vi "Vision Processing.vi"(4 "error in (no error)":errorcluster, 7 "Image Size":T1=enum."320x240") -> ()   [LabVIEW 2015]
doc: "This VI runs in parallel to other tasks. It gets images from the camera, processes them for color or shape and use that information to affect robot behavior."
uses:
  Support Vision Code/Camera Types.ctl
  <vilib>/Rock Robotics/WPI/Camera/WPI_CameraImageSize.ctl
  <userlib>/836-Library/System/QCP Support Code/QCP_Get_DBL.vi
  <userlib>/836-Library/System/QCP Support Code/QCP_Get_STR.vi
  <vilib>/Rock Robotics/Network Tables/NT Read Boolean.vi
  <userlib>/836-Library/System/QCP Support Code/QCP_Set_DBL.vi
  <vilib>/Rock Robotics/Network Tables/NT Write String.vi
  <vilib>/Rock Robotics/Network Tables/NT Write Number.vi
  <vilib>/Rock Robotics/Network Tables/NT Write Boolean.vi
  <vilib>/Rock Robotics/Network Tables/NT Read Number.vi
  <vilib>/Rock Robotics/Network Tables/NT Read String.vi
  Robot Global Data.vi
  <vilib>/vision/NI_Vision_Development_Module.lvlib
panel:
  out "Right Target":dbl
  out "Left Target":dbl
  out "Target Angle":dbl
  in  "Sideways Camera":bool
  in  "Boresight":dbl format="%#_13g"
  out "Found Targets":T2(array[cluster])=[{"Bounding box"={"left"=112.0, "top"=150.0, "right"=139.0, "bottom"=174.0}, "Aspect Ratio"=70.3125, "Area to CH"=96.83972911963883, "X Mask"=77.77777777777779, "Y Mask"=70.83333333333334, "Moment"=69.2156660279794}]
  out "FPS":dbl=5.212996497577636
  out "Qualified Particles":i32=2
  in  "Score Threshold":dbl=70.0
  in  "Aspect Fudge Factor":dbl=1.0
  in  "Min Score Threshold":dbl=75.0
  in  "Camera Type":T3=enum."MS HD3000 square"
  in  "Emphasize Limit Tests":bool
  out "Masked":T4(plugin-control)
  out "Original Image":T4(plugin-control)
  in  "Display Original":bool=TRUE
  out "Sorted Particle Scores":T5(array[cluster])=[{"Rectangle px"={"Numeric"=112.0, "Numeric 2"=150.0, "Numeric 3"=139.0, "Numeric 5"=174.0}, "Aspect Ratio"=70.3125, "Area to CH"=96.83972911963883, "X"=77.77777777777779, "Y"=70.83333333333334, "Moment Factor"=69.2156660279794}] {"Moment Factor" format="%#_3g"; "Aspect Ratio" format="%#_3g"; "Area to CH" format="%#_3g"; "X" format="%#_3g"; "Y" format="%#_3g"}
  out "Detected Targets":T6(array[cluster])=[{"Distance (ft)"=26.324888830153935, "Center"={-0.3966346153846153, -0.35}, "Normalized Rect"={"Numeric"=-0.46153846153846145, "Numeric 2"=-0.25, "Numeric 3"=-0.33173076923076916, "Numeric 5"=-0.44999999999999996}}] {"Normalized Rect"."Numeric 5" format="%#_2g"; "Normalized Rect"."Numeric 3" format="%#_2g"; "Normalized Rect"."Numeric 2" format="%#_2g"; "Normalized Rect"."Numeric" format="%#_2g"}
  in  "LED Color":T7={"Hue"={152.2312396148097, 250.0}, "Sat"={154.82142857142858, 255.0}, "Val"={100.17857142857143, 255.0}} {"Hue" scale=0.0..255.0 scale format="%#_3g"}
  # "Density Profile"
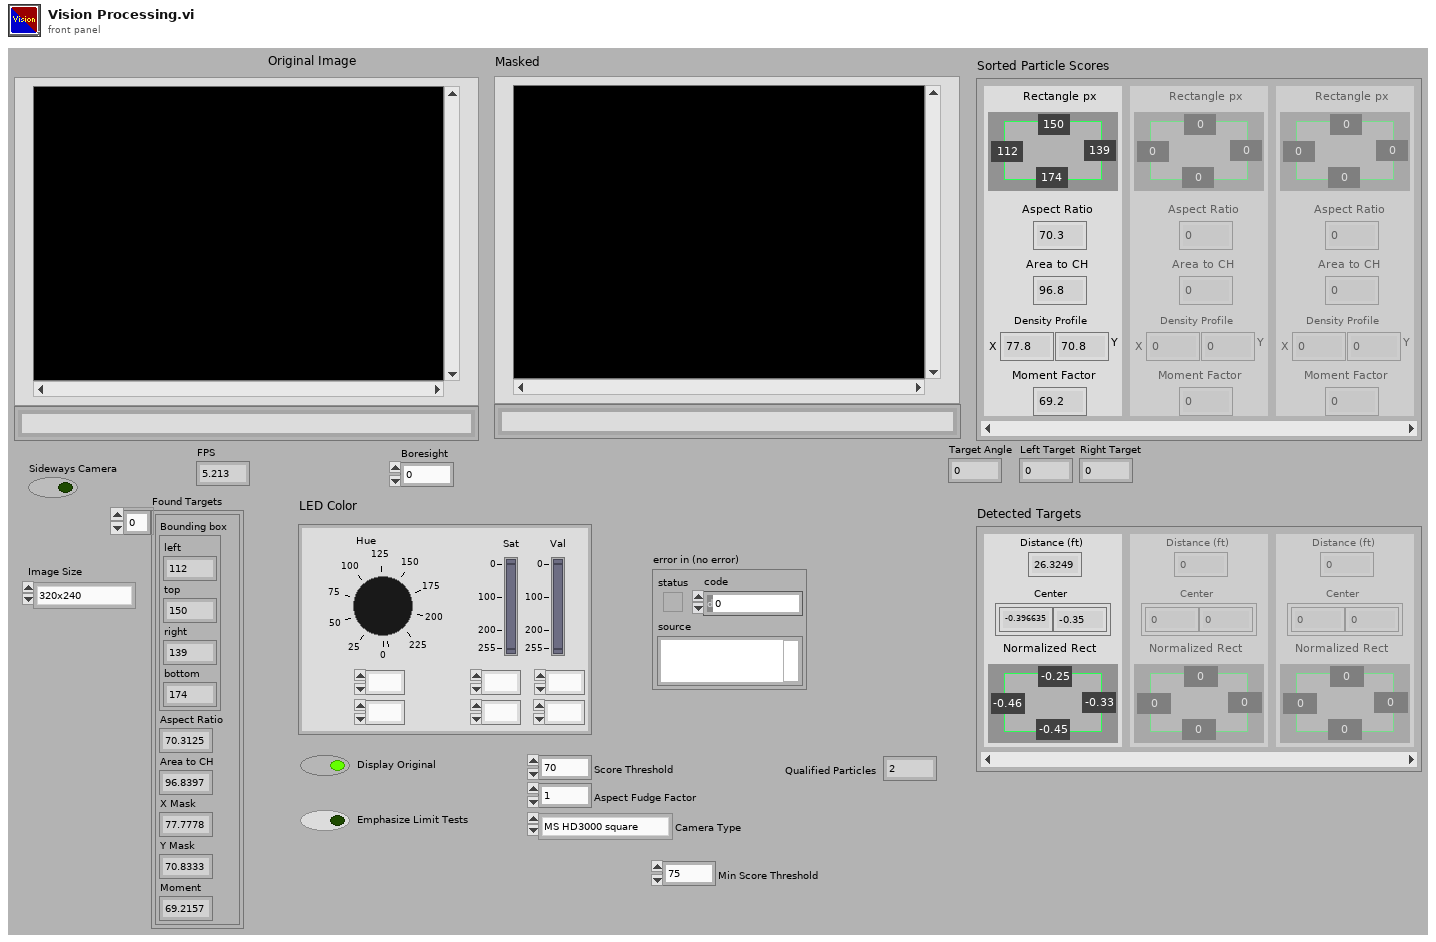
[diagram p1: front panel]
types:
  T1 = typedef "WPI_CameraImageSize.ctl" = enum16{"640x480", "320x240", "160x120", "Custom"}
  T2 = cluster{"Bounding box":cluster{"left":dbl, "top":dbl, "right":dbl, "bottom":dbl}, "Aspect Ratio":dbl, "Area to CH":dbl, "X Mask":dbl, "Y Mask":dbl, "Moment":dbl}[]
  T3 = typedef "Camera Types.ctl" = enum16{"206", "1011", "1013", "MS HD3000 square", "MS HD3000 640x480"}
  T4 = typedef "IMAQ Image.ctl" = refnum<image>
  T5 = cluster{"Rectangle px":cluster{"Numeric":dbl, "Numeric 2":dbl, "Numeric 3":dbl, "Numeric 5":dbl}, "Aspect Ratio":dbl, "Area to CH":dbl, "X":dbl, "Y":dbl, "Moment Factor":dbl}[]
  T6 = cluster{"Distance (ft)":dbl, "Center":cluster{dbl, dbl}, "Normalized Rect":cluster{"Numeric":dbl, "Numeric 2":dbl, "Numeric 3":dbl, "Numeric 5":dbl}}[]
  T7 = cluster{"Hue":cluster{dbl, dbl}, "Sat":cluster{dbl, dbl}, "Val":cluster{dbl, dbl}}
  T8 = typedef "Particle Parameters" = i32
  T9 = typedef "Image Type" = u32
  T10 = typedef "QCP Data Block.ctl" = refnum<data-value>
  T11 = typedef "WPI_CameraDevRef.ctl" = cluster{"Camera Address":string, "CameraStatus":errorcluster}
  T12 = cluster{cluster{"Value Out":dbl, "Value Out":dbl}, cluster{"Value Out":dbl, "Value Out":dbl}, cluster{"Value Out":dbl, "Value Out":dbl}}
  T13 = cluster{"Rectangle":cluster{"Numeric":dbl, "Numeric 2":dbl, "Numeric 3":dbl, "Numeric 5":dbl}, "L":dbl, "Area to CH":dbl, "X":dbl, "Y":dbl, "Moment Factor":dbl}[]
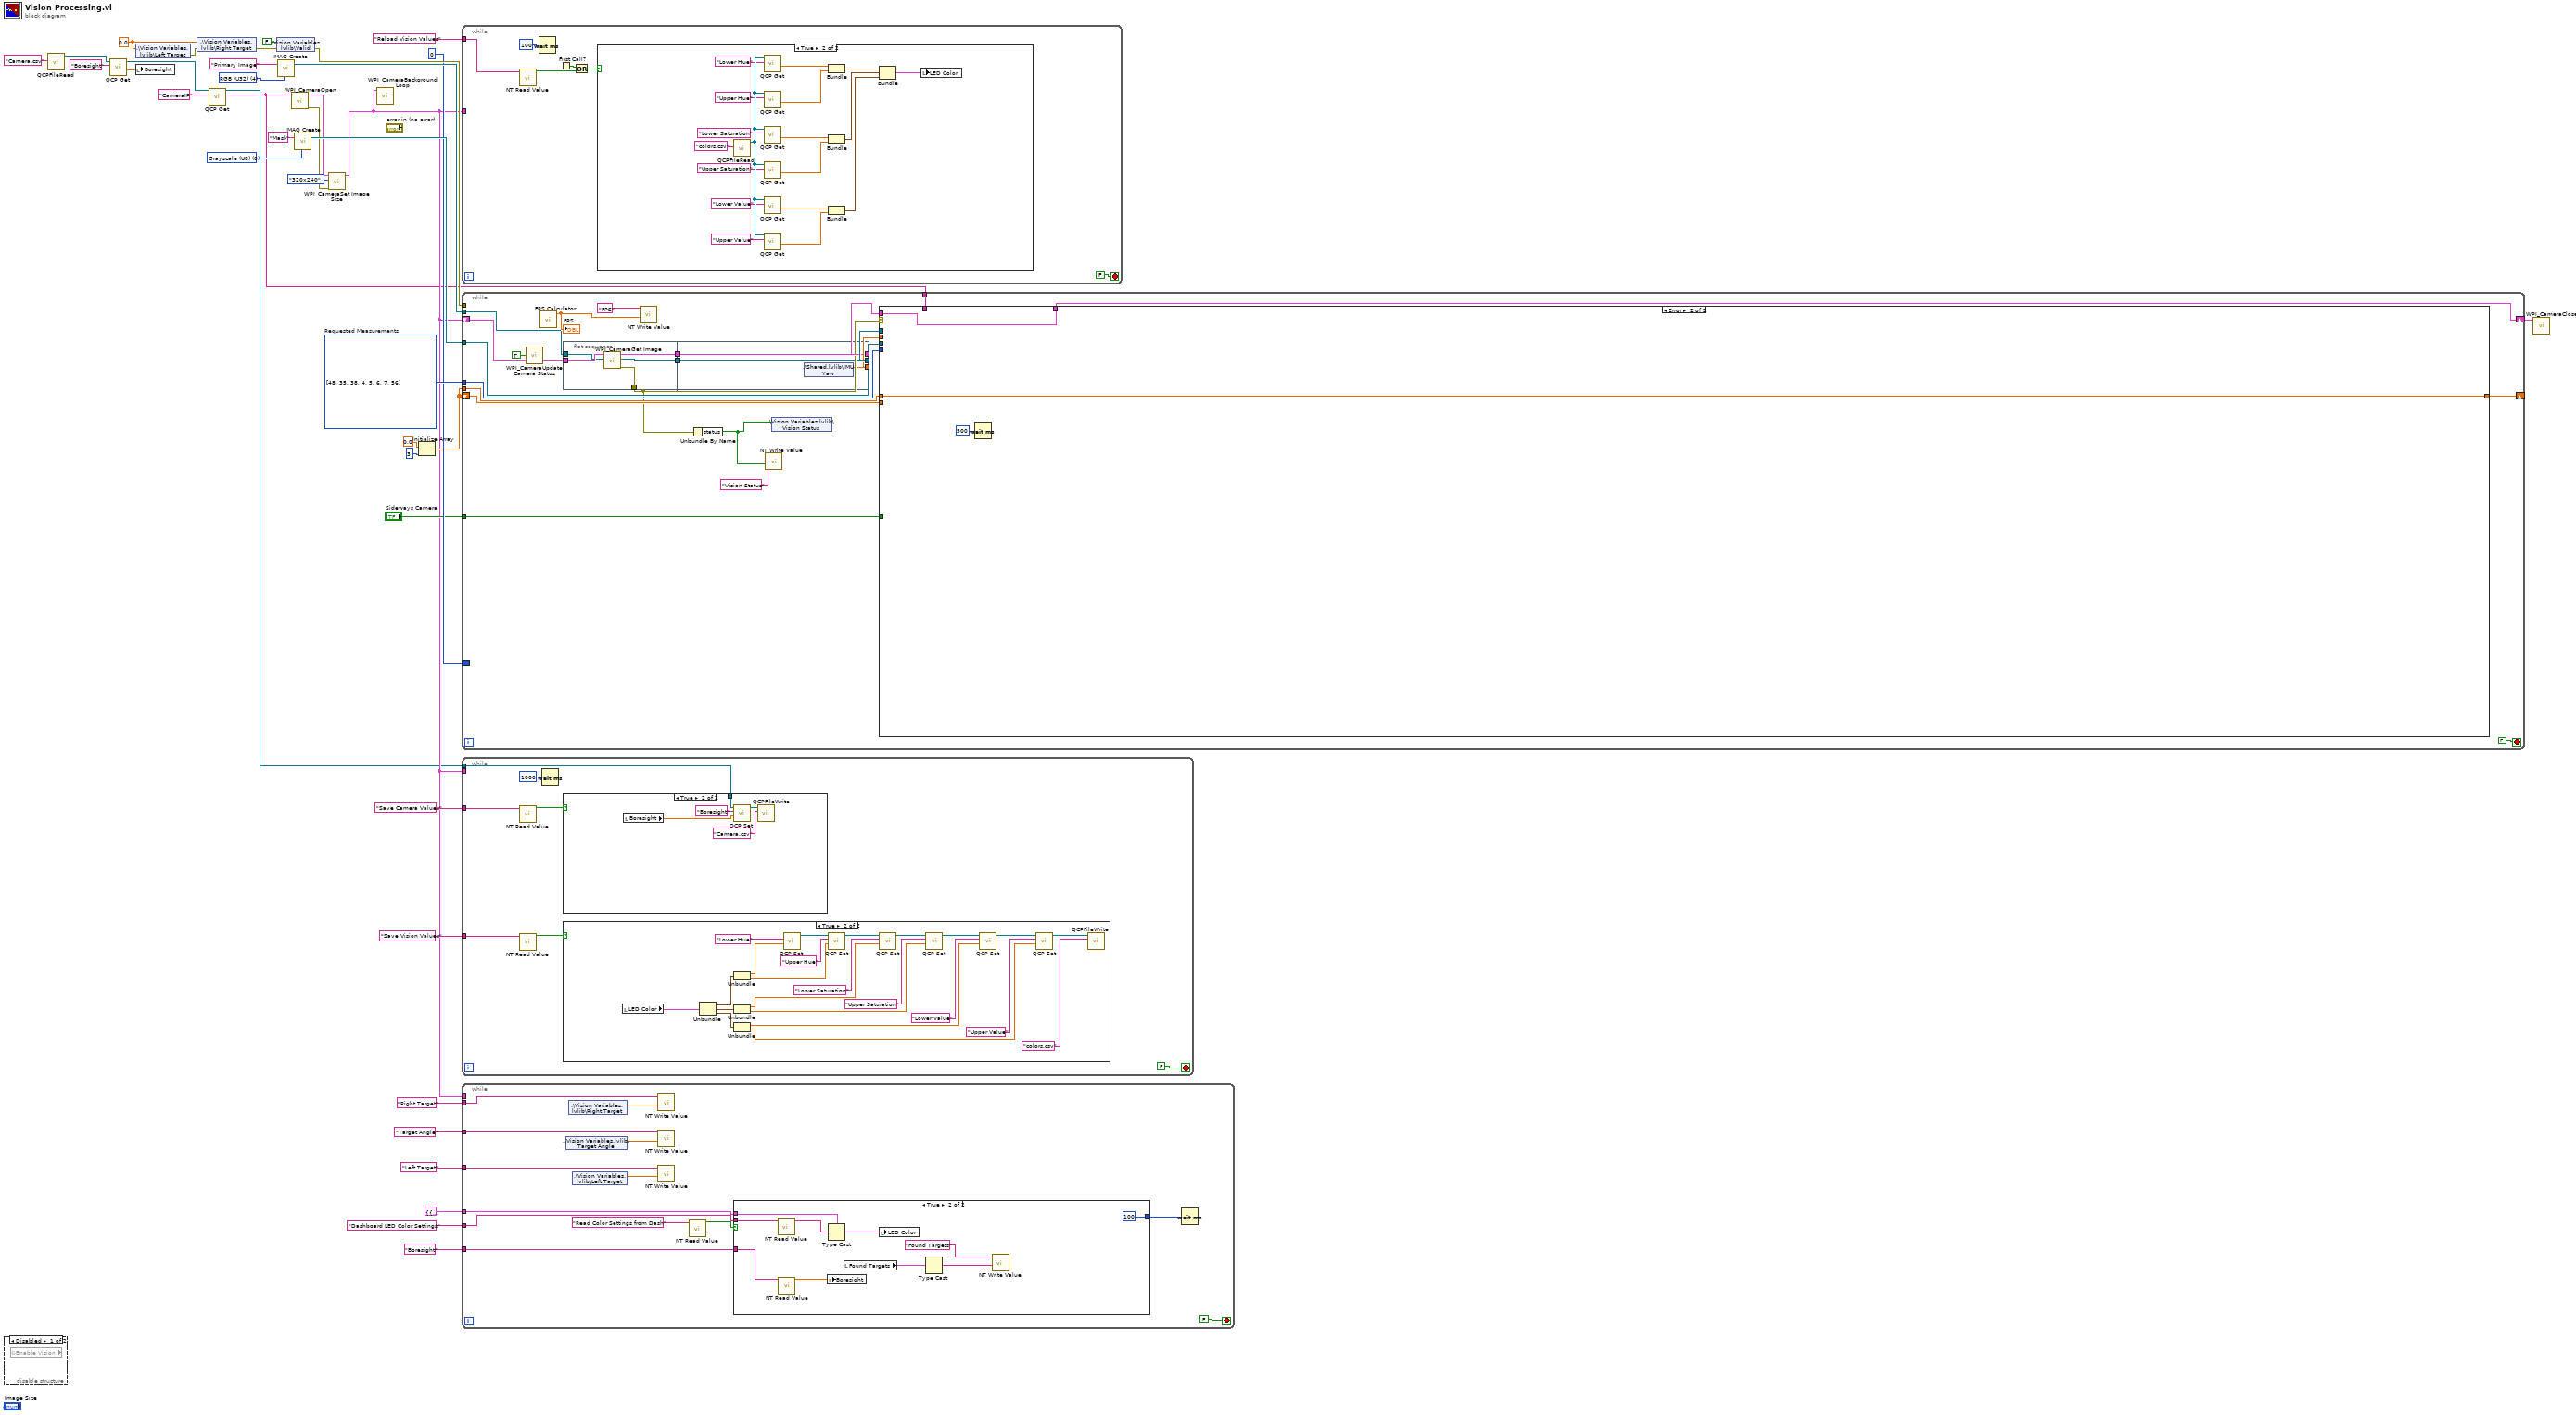
[diagram p0: block diagram]
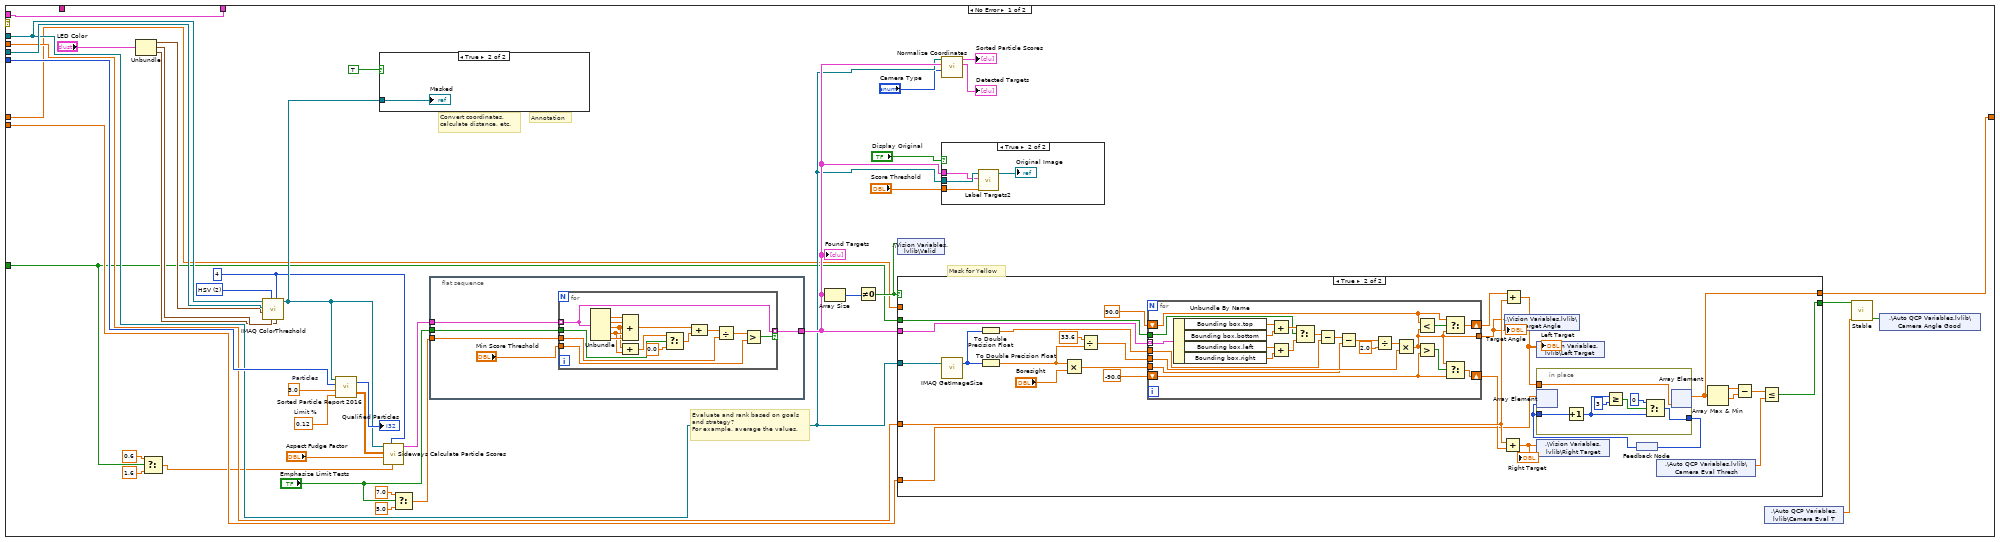
[diagram p3: hidden frame]
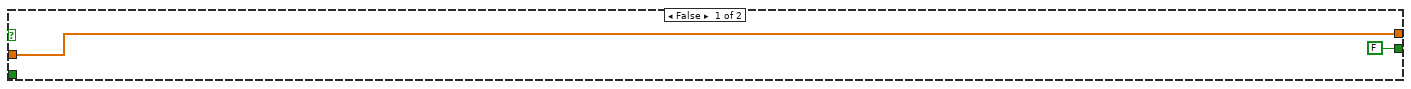
[diagram p6: hidden frame]
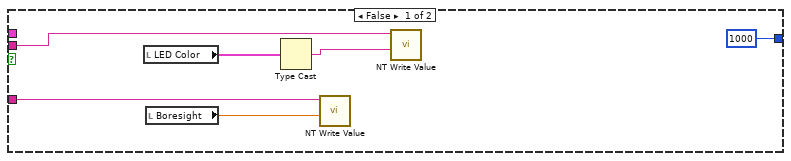
[diagram p7: hidden frame]
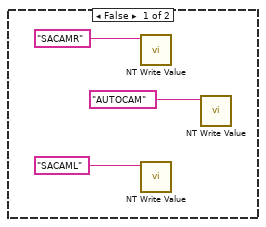
[diagram p8: hidden frame]
diagram:
  w16 = T8[] [48, 35, 38, 4, 5, 6, 7, 56] items=["Center of Mass X", "Center of Mass Y", "First Pixel X", "First Pixel Y", "Bounding Rect Left", "Bounding Rect Top", "Bounding Rect Right", "Bounding Rect Bottom", "Max Feret Diameter Start X", "Max Feret Diameter Start Y", "Max Feret Diameter End X", "Max Feret Diameter End Y", "Max Horiz. Segment Length Left", "Max Horiz. Segment Length Right", "Max Horiz. Segment Length Row", "-", "Bounding Rect Width", "Bounding Rect Height", "Bounding Rect Diagonal", "Perimeter", "Convex Hull Perimeter", "Holes' Perimeter", "Max Feret Diameter", "Equivalent Ellipse Major Axis", "Equivalent Ellipse Minor Axis", "Equivalent Ellipse Minor Axis (Feret)", "Equivalent Rect Long Side", "Equivalent Rect Short Side", "Equivalent Rect Diagonal", "Equivalent Rect Short Side (Feret)", "Average Horiz. Segment Length", "Average Vert. Segment Length", "Hydraulic Radius", "Waddel Disk Diameter", "-", "Area", "Holes' Area", "Particle & Holes' Area", "Convex Hull Area", "Image Area", "-", "Number of Holes", "Number of Horiz. Segments", "Number of Vert. Segments", "-", "Orientation", "Max Feret Diameter Orientation", "-", "% Area/Image Area", "% Area/(Particle & Holes' Area)", "Ratio of Equivalent Ellipse Axes", "Ratio of Equivalent Rect Sides", "-", "Elongation Factor", "Compactness Factor", "Heywood Circularity Factor", "Type Factor", "-", "Sum X", "Sum Y", "Sum XX", "Sum XY", "Sum YY", "Sum XXX", "Sum XXY", "Sum XYY", "Sum YYY", "-", "Moment of Inertia XX", "Moment of Inertia XY", "Moment of Inertia YY", "Moment of Inertia XXX", "Moment of Inertia XXY", "Moment of Inertia XYY", "Moment of Inertia YYY", "Norm. Moment of Inertia XX", "Norm. Moment of Inertia XY", "Norm. Moment of Inertia YY", "Norm. Moment of Inertia XXX", "Norm. Moment of Inertia XXY", "Norm. Moment of Inertia XYY", "Norm. Moment of Inertia YYY", "Hu Moment 1", "Hu Moment 2", "Hu Moment 3", "Hu Moment 4", "Hu Moment 5", "Hu Moment 6", "Hu Moment 7"]  # Requested Measurements
  w27 = 0.0 ("Left Target")
  w35 = T9 0 items=["Grayscale (U8)", "Grayscale (I16)", "Grayscale (SGL)", "Complex (CSG)", "RGB (U32)", "HSL (U32)", "RGB (U64)", "Grayscale (U16)"] ("Image Type")
  w38 = T9 4 items=["Grayscale (U8)", "Grayscale (I16)", "Grayscale (SGL)", "Complex (CSG)", "RGB (U32)", "HSL (U32)", "RGB (U64)"] ("Image Type")
  n1 = disable-structure shown="Disabled" {
    frame Disabled {
      n2 = global read "Robot Global Data.vi" "Enable Vision"() -> ()  [unwired: 1 out]
    }
    frame Enabled {
    }
  }
  n3 = call <userlib>:"QCPFileRead.vi"("File Path"="Camera.csv") -> ("QCP Data Block Out"=w15:T10)  [unwired: 9 in, 1 out]
  n4 = call-poly <userlib>:"QCP Get.vi"("QCP Data Block In"=w15, "QCP Name"="Boresight") -> ("QCP Data Block Out"=w8:T10, "Value Out"=w21:dbl)  [unwired: 6 in, 1 out]
  n5 = shared-variable ".\\Vision Variables.lvlib\\Left Target"(w27) -> (error out=w18:errorcluster)  [unwired: 1 in]
  n6 = local write "Boresight"(w21) -> ()
  n7 = shared-variable ".\\Vision Variables.lvlib\\Right Target"(w27, error in=w18) -> (error out=w17:errorcluster)
  n8 = call-poly <userlib>:"QCP Get.vi"("QCP Data Block In"=w8, "QCP Name"="CameraIP") -> ("QCP Data Block Out"=w2:T10, "Value Out"=w1:string)  [unwired: 6 in, 1 out]
  n9 = shared-variable ".\\Vision Variables.lvlib\\Valid"(FALSE ("Valid"), error in=w17) -> (error out=w19:errorcluster)
  n10 = call "IMAQ Create"("Image Name"="Primary Image", "Image Type"=w38) -> ("New Image"=w36:T4)  [unwired: 2 in, 2 out]
  n11 = call <vilib>:"WPI_CameraOpen.vi"("Camera Address"=w1) -> ("error out"=w4:errorcluster, "CameraDevRef"=w6:T11)  [unwired: 9 in]
  n12 = call "IMAQ Create"("Image Name"="Mask", "Image Type"=w35) -> ("New Image"=w33:T4)  [unwired: 2 in, 2 out]
  n13 = call <vilib>:"WPI_CameraSet Image Size.vi"("error in (no error)"=w4, "Image Size"=WPI_CameraImageSize."320x240", "CameraDevRef"=w6) -> ("CameraDevRef Out"=w5:T11)  [unwired: 7 in, 1 out]
  n14 = call <vilib>:"WPI_CameraBackground Loop.vi"("CameraDevRef"=w5) -> ()  [unwired: 11 in]
  n15 = Initialize Array(0.0, 3 ("dimension size")) -> (w10:dbl[])
  n16 = while {
    tunnel: w5 -> [_]
    tunnel: "Reload Vision Values" ("Name") -> [w40]
    stop <- FALSE stop-if-true
    n17 = call-poly <vilib>:"NT Read Value.vi"("Name"=w40) -> ("Boolean"=w42:bool)  [unwired: 9 in, 1 out]
    n18 = Wait (ms)(milliseconds to wait=u32 100) -> ()  [unwired: 1 out]
    n19 = First Call?() -> (First Call?: T/F=w43:bool)
    n20 = Or(x=w43, y=w42) -> (x .or. y?=w41:bool)
    n21 = case shown="True" w41 {
      frame False {
      }
      frame True {
        n22 = call <userlib>:"QCPFileRead.vi"("File Path"="colors.csv") -> ("QCP Data Block Out"=w63:T10)  [unwired: 9 in, 1 out]
        n23 = call-poly <userlib>:"QCP Get.vi"("QCP Data Block In"=w63, "QCP Name"="Lower Hue") -> ("Value Out"=w55:dbl)  [unwired: 6 in, 2 out]
        n24 = call-poly <userlib>:"QCP Get.vi"("QCP Data Block In"=w63, "QCP Name"="Upper Hue") -> ("Value Out"=w54:dbl)  [unwired: 6 in, 2 out]
        n25 = call-poly <userlib>:"QCP Get.vi"("QCP Data Block In"=w63, "QCP Name"="Lower Saturation") -> ("Value Out"=w52:dbl)  [unwired: 6 in, 2 out]
        n26 = call-poly <userlib>:"QCP Get.vi"("QCP Data Block In"=w63, "QCP Name"="Upper Saturation") -> ("Value Out"=w51:dbl)  [unwired: 6 in, 2 out]
        n27 = call-poly <userlib>:"QCP Get.vi"("QCP Data Block In"=w63, "QCP Name"="Lower Value") -> ("Value Out"=w48:dbl)  [unwired: 6 in, 2 out]
        n28 = call-poly <userlib>:"QCP Get.vi"("QCP Data Block In"=w63, "QCP Name"="Upper Value") -> ("Value Out"=w47:dbl)  [unwired: 6 in, 2 out]
        n29 = Bundle("Value Out"=w55, "Value Out"=w54) -> (w53:cluster{"Value Out":dbl, "Value Out":dbl})  [unwired: 1 in]
        n30 = Bundle("Value Out"=w52, "Value Out"=w51) -> (w50:cluster{"Value Out":dbl, "Value Out":dbl})  [unwired: 1 in]
        n31 = Bundle("Value Out"=w48, "Value Out"=w47) -> (w49:cluster{"Value Out":dbl, "Value Out":dbl})  [unwired: 1 in]
        n32 = Bundle(w53, w50, w49) -> (w46:T12)  [unwired: 1 in]
        n33 = local write "LED Color"(w46) -> ()
      }
    }
  }
  n34 = while {
    shift-right: [w69] -> w32
    shift-left: w5 -> [w71]
    tunnel: w36 -> [w83]
    tunnel: w33 -> [w76]
    tunnel: w16 -> [w82]
    tunnel: w19 -> [_]
    border: 0 -> [_]
    shift-right: [w75] -> _
    shift-left: w10 -> [w74]
    tunnel: w10 -> [w73]
    tunnel: "Sideways Camera" -> [w72]
    tunnel: w1 -> [w68]
    stop <- FALSE stop-if-true
    n35 = call <vilib>:"WPI_CameraUpdate Camera Status.vi"("CameraDevRef In"=w71, "Enable Vision"=TRUE) -> ("CameraDevRef Out"=w81:T11)  [unwired: 3 in]
    n36 = call <userlib>:"FPS Calculator.vi"() -> ("FPS"=w85:dbl)  [unwired: 11 in]
    "FPS" <- w85
    n37 = flat-sequence {
      tunnel: w81 -> [w220]
      tunnel: w83 -> [w219]
      tunnel: [w218] -> w80
      tunnel: [w217] -> w79
      tunnel: [w216] -> w67
      tunnel: [w222] -> w78
      tunnel: [w223] -> w70
      tunnel: w80 -> [w223]
      tunnel: w79 -> [w222]
      tunnel: [w221] -> w77
      frame #0 {
        n38 = call <vilib>:"WPI_CameraGet Image.vi"("Image"=w219, "CameraDevRef"=w220) -> ("error out"=w216:errorcluster, "Image Out"=w217:T4, "CameraDevRef Out"=w218:T11)  [unwired: 7 in]
      }
      frame #1 {
        n39 = shared-variable ".\\Shared.lvlib\\IMU Yaw"() -> (w221:dbl)  [unwired: 1 in, 1 out]
      }
    }
    n40 = call-poly <vilib>:"NT Write Value.vi"("Numeric"=w85, "Name"="FPS") -> ()  [unwired: 9 in, 1 out]
    n41 = Unbundle By Name(w67) -> ("status"=w65:bool)
    n42 = call-poly <vilib>:"NT Write Value.vi"("Boolean"=w65, "Name"="Vision Status") -> ()  [unwired: 9 in, 1 out]
    n43 = shared-variable ".\\Vision Variables.lvlib\\Vision Status"(w65) -> ()  [unwired: 1 in, 1 out]
    n44 = case shown="Error" w67 {
      tunnel: w76 -> [w127 _]
      tunnel: w82 -> [w123 _]
      tunnel: w78 -> [w107 _]
      tunnel: w77 -> [w106 _]
      tunnel: w74 -> [w102 _]
      tunnel: [w100 w215] -> w75
      tunnel: w73 -> [w99 w215]
      tunnel: w72 -> [w94 _]
      tunnel: w70 -> [w87 w214]
      tunnel: [w87 w214] -> w69
      tunnel: w68 -> [_ _]
      frame No Error {
        w111 = 4 ("Replace Value")
        w119 = u16 2 items=["RGB", "HSL", "HSV", "HSI"] ("Color Mode")
        w120 = 0.12  # Limit %
        w122 = 3.0  # Particles
        # "Convert coordinates,\ncalculate distance, etc."
        # "Annotation"
        # "Evaluate and rank based on goals\nand strategy?\nFor example, average the values."
        # "Mask for Yellow"
        n45 = Unbundle("LED Color") -> ("Hue"=w126:cluster{dbl, dbl}, "Sat"=w125:cluster{dbl, dbl}, "Val"=w124:cluster{dbl, dbl})
        n46 = Select(t=0.6 ("Expected Aspect Ratio"), s=w94, f=1.6) -> (s? t:f=w96:dbl)
        n47 = call "IMAQ ColorThreshold"("Blue or Luma or Val or Inten Range"=w124, "Replace Value"=w111, "Green or Sat Range"=w125, "Color Mode"=w119, "Red or Hue Range"=w126, "Image Dst"=w127, "Image Src"=w107) -> ("Image Dst Out"=w118:T4)  [unwired: 3 in, 1 out]
        n48 = call "Sorted Particle Report 2016.vi"("Min Area Size %"=w120, "Particle Count Limit"=w122, "Pixel Measurements"=w123, "Image in"=w118) -> ("Sorted Data"=w117:dbl[][], "Particles"=→"Qualified Particles":i32)
        n49 = case shown="True" TRUE ("Display Mask") {
          tunnel: w118 -> [_ w132]
          frame False {
          }
          frame True {
            "Masked" <- w132
          }
        }
        n50 = call "Sideways Calculate Particle Scores.vi"("Expected Aspect Ratio"=w96, "Pixel Value"=w111, "Aspect Fudge Factor"="Aspect Fudge Factor", "Sorted Data"=w117, "Image in"=w118) -> ("Scores"=w115:T2)  [unwired: 6 in]
        n51 = Select(t=7.0, s="Emphasize Limit Tests", f=5.0) -> (s? t:f=w112:dbl)
        n52 = flat-sequence {
          tunnel: w115 -> [w137]
          tunnel: w112 -> [w135]
          tunnel: [w133] -> w109
          tunnel: "Emphasize Limit Tests" -> [w136]
          frame #0 {
            n53 = for {
              tunnel: w137 -> [w151] mode=indexing
              tunnel: [w151] -> w133 mode=indexing if=w150
              tunnel: w135 -> [w148]
              tunnel: "Min Score Threshold" -> [w147]
              tunnel: w136 -> [w140]
              n54 = Unbundle(w151) -> ("Aspect Ratio"=w153:dbl, "Area to CH"=w152:dbl, "X Mask"=w142:dbl, "Y Mask"=w143:dbl, "Moment"=w144:dbl)  [unwired: 1 out]
              n55 = Compound Arithmetic op=ADD(w153, w152, w142, w143, w144) -> (w146:dbl)
              n56 = Compound Arithmetic op=ADD(w142, w143) -> (w141:dbl)
              n57 = Select(t=w141, s=w140, f=0.0) -> (s? t:f=w139:dbl)
              n58 = Compound Arithmetic op=ADD(w146, w139) -> (w145:dbl)
              n59 = Divide(x=w145, y=w148) -> (x/y=w149:dbl)
              n60 = Greater?(x=w149, y=w147) -> (0:w150:bool)
            }
          }
        }
        n61 = Array Size(array=w109) -> (size(s)=w108:i32)
        n62 = Not Equal To 0?(x=w108) -> (x != 0?=w104:bool)
        n63 = shared-variable ".\\Vision Variables.lvlib\\Valid"(w104) -> ()  [unwired: 1 in, 1 out]
        n64 = case shown="True" w104 {
          tunnel: w109 -> [_ w182]
          tunnel: w106 -> [_ w181]
          tunnel: w107 -> [_ w174]
          tunnel: w102 -> [_ w166]
          tunnel: [FALSE w158] -> w101
          tunnel: [w154 w157] -> w100
          tunnel: w99 -> [w154 _]
          tunnel: w94 -> [_ w156]
          frame False {
          }
          frame True {
            n65 = call "IMAQ GetImageSize"("Image"=w174) -> ("Y Resolution"=w171:i32)  [unwired: 3 in, 2 out]
            n66 = To Double Precision Float(number=w171) -> (double precision float=w173:dbl)
            n67 = To Double Precision Float(number=w171) -> (double precision float=w169:dbl)
            n68 = Multiply(x=w169, y="Boresight") -> (x*y=w168:dbl)
            n69 = Divide(x=33.6, y=w169) -> (x/y=w175:dbl)
            n70 = for {
              tunnel: w182 -> [w212] mode=indexing
              tunnel: w173 -> [w209]
              tunnel: w175 -> [w208]
              shift-right: [w205] -> w177
              shift-left: -90.0 -> [w203]
              shift-right: [w204] -> w178
              shift-left: 90.0 -> [w200]
              tunnel: w168 -> [w198]
              tunnel: [w196] -> w167
              tunnel: w156 -> [w191]
              n71 = Unbundle By Name(w212) -> ("Bounding box.top"=w211:dbl, "Bounding box.bottom"=w210:dbl, "Bounding box.left"=w194:dbl, "Bounding box.right"=w195:dbl)
              n72 = Add(x=w211, y=w210) -> (x+y=w193:dbl)
              n73 = Add(x=w194, y=w195) -> (x+y=w192:dbl)
              n74 = Select(t=w193, s=w191, f=w192) -> (s? t:f=w190:dbl)
              n75 = Subtract(x=w190, y=w209) -> (x-y=w199:dbl)
              n76 = Subtract(x=w199, y=w198) -> (x-y=w197:dbl)
              n77 = Divide(x=w197, y=2.0) -> (x/y=w201:dbl)
              n78 = Multiply(x=w201, y=w208) -> (x*y=w196:dbl)
              n79 = Less?(x=w200, y=w196) -> (x < y?=w207:bool)
              n80 = Greater?(x=w196, y=w203) -> (0:w206:bool)
              n81 = Select(t=w200, s=w207, f=w196) -> (s? t:f=w204:dbl)
              n82 = Select(t=w196, s=w206, f=w203) -> (s? t:f=w205:dbl)
            }
            "Target Angle" <- w167
            n83 = Add(x=w181, y=w177) -> (x+y=w172:dbl)
            "Right Target" <- w172
            n84 = Add(x=w178, y=w181) -> (x+y=w165:dbl)
            "Left Target" <- w165
            n85 = shared-variable ".\\Vision Variables.lvlib\\Target Angle"(w167) -> ()  [unwired: 1 in, 1 out]
            n86 = shared-variable ".\\Vision Variables.lvlib\\Left Target"(w165) -> ()  [unwired: 1 in, 1 out]
            n87 = shared-variable ".\\Vision Variables.lvlib\\Right Target"(w172) -> ()  [unwired: 1 in, 1 out]
            n88 = feedback #1() -> (w164:i32)
            n89 = in-place {
              in-place-border: w165 -> [w189]
              in-place-border: w164 -> [w188]
              in-place-border: [w183] -> w163
              n90 = in-place-array #2(w166, w164) -> ()  [unwired: 1 out]
              n91 = Increment(x=w188) -> (x+1=w185:i32)
              n92 = Greater Or Equal?(x=w185, y=3) -> (x >= y?=w186:bool)
              n93 = Select(t=0, s=w186, f=w185) -> (s? t:f=w183:i32)
              n94 = in-place-array #2(w189) -> (w157:dbl[])  [unwired: 1 out]
            }
            n95 = feedback-in #1(w163) -> ()
            n96 = shared-variable ".\\Auto QCP Variables.lvlib\\Camera Eval Thresh"() -> (w159:dbl)  [unwired: 1 in, 1 out]
            n97 = Array Max & Min(array=w157) -> (max value=w162:dbl, min value=w161:dbl)  [unwired: 2 out]
            n98 = Subtract(x=w162, y=w161) -> (x-y=w160:dbl)
            n99 = Less Or Equal?(x=w160, y=w159) -> (x <= y?=w158:bool)
          }
        }
        n100 = call "Normalize Coordinates.vi"("Camera Type"="Camera Type", "Targets"=w109, "Image in"=w107) -> ("Found Targets"=→"Detected Targets":T6, "Sorted Scores"=→"Sorted Particle Scores":T13)  [unwired: 7 in]
        n101 = case shown="True" "Display Original" {
          tunnel: w107 -> [_ w131]
          tunnel: w109 -> [_ w129]
          tunnel: "Score Threshold" -> [_ w128]
          frame False {
          }
          frame True {
            n102 = call "Label Targets2.vi"("Score Threshold"=w128, "Targets"=w129, "Image in"=w131) -> ("Image out"=→"Original Image":T4)  [unwired: 8 in]
          }
        }
        n103 = shared-variable ".\\Auto QCP Variables.lvlib\\Camera Eval T"() -> (w103:dbl)  [unwired: 1 in, 1 out]
        n104 = call <userlib>:"Stable.vi"("Eval Period (sec)"=w103, "Signal Input"=w101) -> ("Stable"=w98:bool)  [unwired: 9 in]
        n105 = shared-variable ".\\Auto QCP Variables.lvlib\\Camera Angle Good"(w98) -> ()  [unwired: 1 in, 1 out]
        "Found Targets" <- w109
      }
      frame Error {
        n106 = Wait (ms)(milliseconds to wait=u32 500) -> ()  [unwired: 1 out]
      }
    }
  }
  n107 = while {
    tunnel: w5 -> [_]
    tunnel: "Save Camera Values" ("Name") -> [w226]
    tunnel: "Save Vision Values" ("Name") -> [w225]
    tunnel: w2 -> [w224]
    stop <- FALSE stop-if-true
    n108 = call-poly <vilib>:"NT Read Value.vi"("Name"=w226) -> ("Boolean"=w227:bool)  [unwired: 9 in, 1 out]
    n109 = call-poly <vilib>:"NT Read Value.vi"("Name"=w225) -> ("Boolean"=w228:bool)  [unwired: 9 in, 1 out]
    n110 = Wait (ms)(milliseconds to wait=u32 1000) -> ()  [unwired: 1 out]
    n111 = case shown="True" w227 {
      tunnel: w224 -> [_ w234]
      frame False {
        n112 = call-poly <vilib>:"NT Write Value.vi"("Name"="SACAMR") -> ()  [unwired: 10 in, 1 out]
        n113 = call-poly <vilib>:"NT Write Value.vi"("Name"="SACAML") -> ()  [unwired: 10 in, 1 out]
        n114 = call-poly <vilib>:"NT Write Value.vi"("Name"="AUTOCAM") -> ()  [unwired: 10 in, 1 out]
      }
      frame True {
        n115 = local read "Boresight"() -> (w236:dbl)
        n116 = call-poly <userlib>:"QCP Set.vi"("QCP Data Block In"=w234, "QCP Name"="Boresight", "Value In"=w236) -> ("QCP Data Block Out"=w235:T10)  [unwired: 7 in]
        n117 = call <userlib>:"QCPFileWrite.vi"("File Path"="Camera.csv", "QCP Data Block In"=w235) -> ()  [unwired: 8 in, 2 out]
      }
    }
    n118 = case shown="True" w228 {
      frame False {
      }
      frame True {
        n119 = local read "LED Color"() -> (w248:T7)
        n120 = Unbundle(w248) -> ("Hue"=w247:cluster{dbl, dbl}, "Sat"=w246:cluster{dbl, dbl}, "Val"=w245:cluster{dbl, dbl})
        n121 = Unbundle(w247) -> (w240:dbl, w239:dbl)
        n122 = Unbundle(w246) -> (w242:dbl, w241:dbl)
        n123 = Unbundle(w245) -> (w244:dbl, w243:dbl)
        n124 = call-poly <userlib>:"QCP Set.vi"("QCP Name"="Lower Hue", "Value In"=w240) -> ("QCP Data Block Out"=w253:T10)  [unwired: 8 in]
        n125 = call-poly <userlib>:"QCP Set.vi"("QCP Data Block In"=w253, "QCP Name"="Upper Hue", "Value In"=w239) -> ("QCP Data Block Out"=w254:T10)  [unwired: 7 in]
        n126 = call-poly <userlib>:"QCP Set.vi"("QCP Data Block In"=w254, "QCP Name"="Lower Saturation", "Value In"=w242) -> ("QCP Data Block Out"=w252:T10)  [unwired: 7 in]
        n127 = call-poly <userlib>:"QCP Set.vi"("QCP Data Block In"=w252, "QCP Name"="Upper Saturation", "Value In"=w241) -> ("QCP Data Block Out"=w251:T10)  [unwired: 7 in]
        n128 = call-poly <userlib>:"QCP Set.vi"("QCP Data Block In"=w251, "QCP Name"="Lower Value", "Value In"=w244) -> ("QCP Data Block Out"=w250:T10)  [unwired: 7 in]
        n129 = call-poly <userlib>:"QCP Set.vi"("QCP Data Block In"=w250, "QCP Name"="Upper Value", "Value In"=w243) -> ("QCP Data Block Out"=w249:T10)  [unwired: 7 in]
        n130 = call <userlib>:"QCPFileWrite.vi"("File Path"="colors.csv", "QCP Data Block In"=w249) -> ()  [unwired: 8 in, 2 out]
      }
    }
  }
  n131 = while {
    tunnel: "Dashboard LED Color Settings" ("Name") -> [w271]
    tunnel: T7 {"Hue"={152.2312396148097, 250.0}, "Sat"={154.82142857142858, 255.0}, "Val"={100.17857142857143, 255.0}} ("LED Color") -> [w270]
    tunnel: w5 -> [_]
    tunnel: "Left Target" ("Name") -> [w266]
    tunnel: "Right Target" ("Name") -> [w265]
    tunnel: "Boresight" ("Name") -> [w264]
    tunnel: "Target Angle" ("Name") -> [w262]
    stop <- FALSE stop-if-true
    n132 = shared-variable ".\\Vision Variables.lvlib\\Target Angle"() -> (w263:dbl)  [unwired: 1 in, 1 out]
    n133 = shared-variable ".\\Vision Variables.lvlib\\Right Target"() -> (w267:dbl)  [unwired: 1 in, 1 out]
    n134 = shared-variable ".\\Vision Variables.lvlib\\Left Target"() -> (w268:dbl)  [unwired: 1 in, 1 out]
    n135 = call-poly <vilib>:"NT Write Value.vi"("Numeric"=w267, "Name"=w265) -> ()  [unwired: 9 in, 1 out]
    n136 = call-poly <vilib>:"NT Write Value.vi"("Numeric"=w263, "Name"=w262) -> ()  [unwired: 9 in, 1 out]
    n137 = call-poly <vilib>:"NT Write Value.vi"("Numeric"=w268, "Name"=w266) -> ()  [unwired: 9 in, 1 out]
    n138 = call-poly <vilib>:"NT Read Value.vi"("Name"="Read Color Settings from Dash") -> ("Boolean"=w272:bool)  [unwired: 9 in, 1 out]
    n139 = case shown="True" w272 {
      tunnel: w271 -> [w279 w288]
      tunnel: w270 -> [_ w287]
      tunnel: [u32 1000 ("milliseconds to wait") u32 100 ("milliseconds to wait")] -> w269
      tunnel: w264 -> [w276 w282]
      frame False {
        n140 = local read "LED Color"() -> (w280:T7)
        n141 = local read "Boresight"() -> (w275:dbl)
        n142 = Type Cast(x=w280) -> (*(type *) &x=w278:string)  [unwired: 1 in]
        n143 = call-poly <vilib>:"NT Write Value.vi"("Numeric"=w275, "Name"=w276) -> ()  [unwired: 9 in, 1 out]
        n144 = call-poly <vilib>:"NT Write Value.vi"("String"=w278, "Name"=w279) -> ()  [unwired: 9 in, 1 out]
      }
      frame True {
        n145 = call-poly <vilib>:"NT Read Value.vi"("Name"=w288) -> ("String"=w289:string)  [unwired: 9 in, 1 out]
        n146 = call-poly <vilib>:"NT Read Value.vi"("Name"=w282) -> ("Numeric"=w281:dbl)  [unwired: 9 in, 1 out]
        n147 = local write "Boresight"(w281) -> ()
        n148 = Type Cast(type=w287, x=w289) -> (*(type *) &x=w290:T7)
        n149 = local read "Found Targets"() -> (w286:T2)
        n150 = local write "LED Color"(w290) -> ()
        n151 = Type Cast(x=w286) -> (*(type *) &x=w285:string)  [unwired: 1 in]
        n152 = call-poly <vilib>:"NT Write Value.vi"("String"=w285, "Name"="Found Targets") -> ()  [unwired: 9 in, 1 out]
      }
    }
    n153 = Wait (ms)(milliseconds to wait=w269) -> ()  [unwired: 1 out]
  }
  n154 = call <vilib>:"WPI_CameraClose.vi"("CameraDevRef"=w32) -> ()  [unwired: 1 in, 10 out]
